vi "Elevator Mode Selector.vi"(9 "Manual?":bool, 10 "Semiauto?":bool) -> (2 "Elevator Mode":T1)   [LabVIEW 2017]
uses:
  Common Code/Elevator Mode.ctl
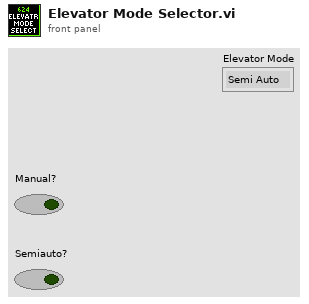
[diagram p1: front panel]
types:
  T1 = typedef "Elevator Mode.ctl" = enum16{"Semi Auto", "Manual", "Auto"}
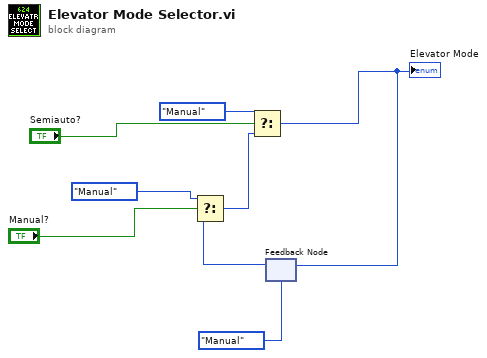
[diagram p0: block diagram]
diagram:
  n1 = feedback #1(Elevator_Mode."Manual" ("Elevator Mode")) -> (w2:T1)
  n2 = Select(t=Elevator_Mode."Manual" ("Elevator Mode"), s="Manual?", f=w2) -> (s? t:f=w4:T1)
  n3 = Select(t=Elevator_Mode."Manual" ("Elevator Mode"), s="Semiauto?", f=w4) -> (s? t:f=w1:T1)
  "Elevator Mode" <- w1
  n4 = feedback-in #1(w1) -> ()
